vi "Decimate mixed channels data (Theo).vi"(9 "Selected Waveform":enum16{"Left graph", "Right graph"}(ring)=enum."Right graph", 10 "waveform":waveform(dbl)={"t0"=timestamp(0 s since 1904-01-01), "dt"=1e-06, "Y"=[]}) -> (0 "multiple tone information":T1(array[cluster])=[{"detected frequency"=59.40457132494078, "detected amplitude"=677.5224683183739, "detected phase (deg)"=-6.85916777032908}, {"detected frequency"=10023.302847711435, "detected amplitude"=302.0949374874943, "detected phase (deg)"=265.4481634375171}, {"detected frequency"=20019.602268100927, "detected amplitude"=136.99007273675608, "detected phase (deg)"=123.98051462950585}, {"detected frequency"=30006.01918128676, "detected amplitude"=20.477000538882503, "detected phase (deg)"=-16.173557072223005}] {"detected phase (deg)" format="%_6g"; "detected amplitude" format="%_6p"; "detected frequency" format="%_6p"}, 2 "output waveform":waveform(dbl))   [LabVIEW 2017]
uses:
  <vilib>/measure/NI_MAPro.lvlib
  <vilib>/express/express analysis/Spectral/XNode/ExpressSpectralMeasurementsBlockNode.xnode
  <vilib>/express/express analysis/Spectral/Block/exnSpectralBlock spectral measurements RMS poly.vi
  <vilib>/express/express analysis/Spectral/Block/exnSpectralBlock spectral measurements RMS WFM.vi
  <vilib>/measure/matone.llb/Extract Multiple Tone Information 1 Chan.vi
panel:
  out "Phase":cluster{"f0":dbl, "df":dbl, "phase":dbl[]}
  out "Measurement Output":cluster{"f0":dbl, "df":dbl, "magnitude":dbl[]}
  in  "Paste copied Excel data column in this box":string="442\n58\n454\n60\n425\n59\n424\n63\n423\n64\n371\n59\n492\n63\n416\n60\n390\n63\n393\n64\n472\n60\n457\n59\n461\n61\n383\n62\n415\n61\n416\n59\n421\n61\n430\n60\n440\n63\n429\n55\n407\n60\n479\n63\n463\n64\n389\n54\n449\n65\n443\n61\n415\n61\n419\n62\n396\n61\n379\n56\n386\n60\n404\n69\n349\n62\n466\n58\n450\n62\n414\n57\n433\n61\n477\n63\n397\n60\n402\n58\n457\n59\n466\n61\n445\n60\n416\n62\n459\n65\n464\n65\n441\n62\n408\n63\n437\n57\n388\n60\n429\n65\n445\n55\n460\n66\n419\n60\n431\n59\n450\n64\n451\n60\n435\n63\n431\n61\n450\n62\n423\n60\n423\n61\n434\n62\n454\n65\n417\n65\n403\n58\n462\n57\n430\n56\n451\n56\n431\n59\n384\n56\n462\n66\n476\n59\n436\n62\n460\n64\n467\n60\n430\n55\n411\n56\n498\n61\n426\n68\n469\n66\n445\n56\n428\n55\n455\n62\n447\n59\n407\n6..."
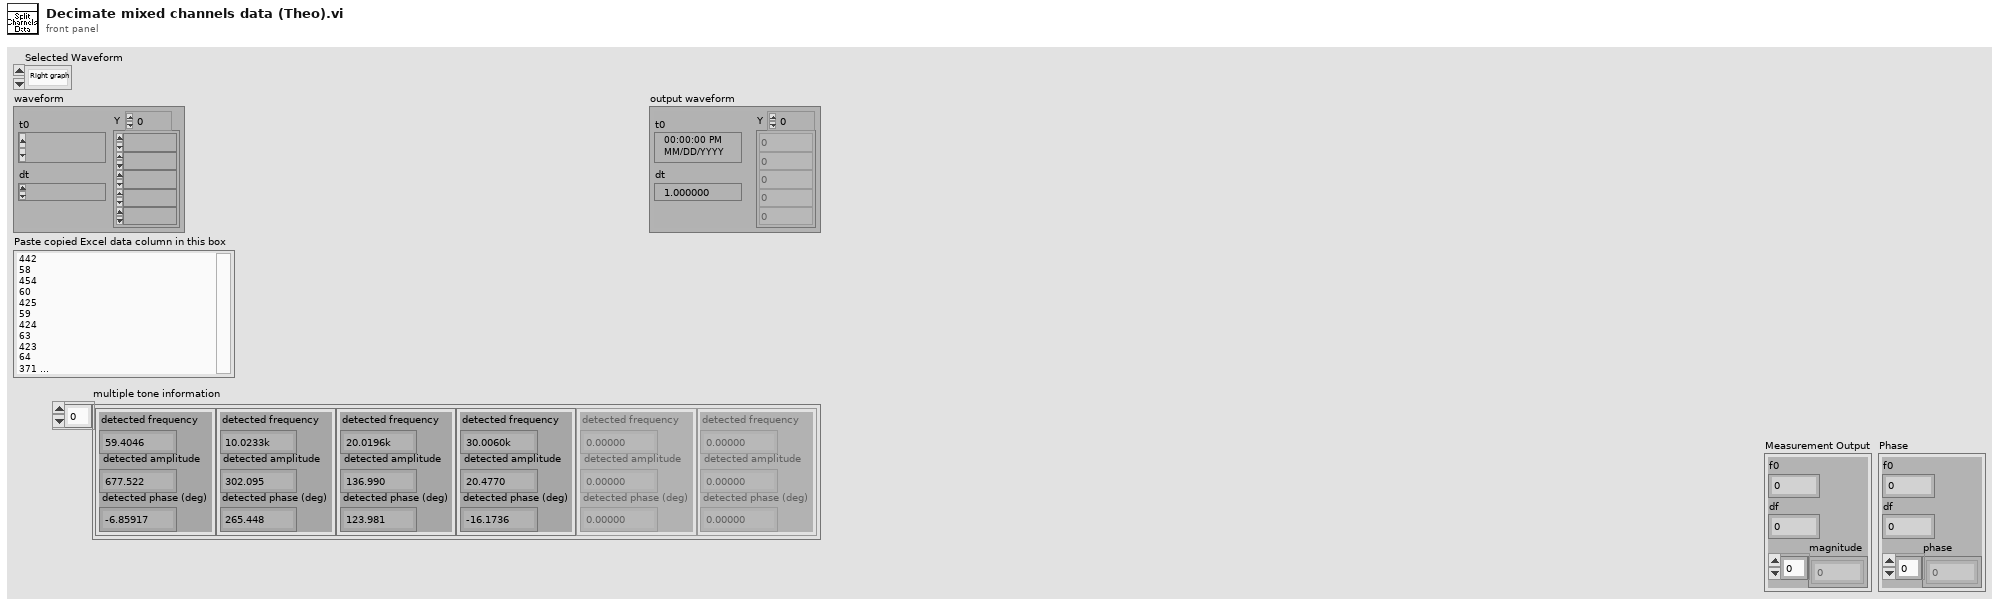
[diagram p1: front panel]
types:
  T1 = cluster{"detected frequency":dbl, "detected amplitude":dbl, "detected phase (deg)":dbl}[]
  T2 = enum32{"none", "input signal", "detected signal", "residual signal"}
  T3 = cluster{"averaging mode":u16, "weighting mode":u16, "number of averages":u32}
  T4 = cluster{"dB On (F)":bool, "unwrap phase (F)":bool, "convert to degree (F)":bool}
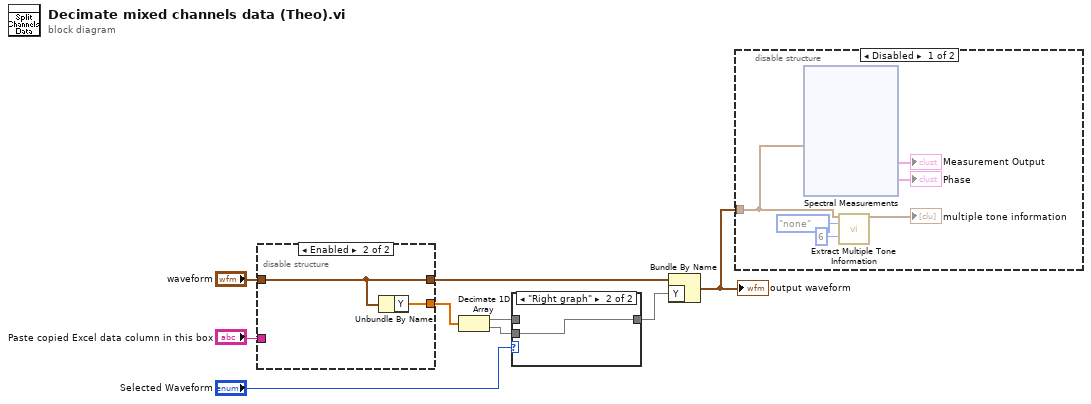
[diagram p0: block diagram]
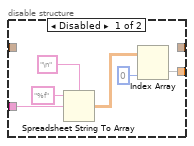
[diagram p4: hidden frame]
diagram:
  n1 = disable-structure shown="Enabled" {
    disable-tunnel: "Paste copied Excel data column in this box" -> [w15 _]
    disable-tunnel: [w10 w17] -> w8
    disable-tunnel: "waveform" -> [_ w16]
    disable-tunnel: [_ w16] -> w5
    frame Disabled {
      n2 = Spreadsheet String To Array(delimiter (Tab)="\n", format string="%f", spreadsheet string=w15) -> (array=w12:dbl[][])  [unwired: 1 in]
      n3 = Index Array(array=w12, index (col)=0 ("disabled index (col)")) -> (element=w10:dbl[])  [unwired: 1 in]
    }
    frame Enabled {
      n4 = Unbundle By Name(w16) -> ("Y"=w17:dbl[])
    }
  }
  n5 = Decimate 1D Array(w8) -> (w4:dbl[], w2:dbl[])
  n6 = case shown="\"Right graph\"" "Selected Waveform" {
    tunnel: w4 -> [w18 _]
    tunnel: [w18 w19] -> w3
    tunnel: w2 -> [_ w19]
    frame "Left graph", Default {
    }
    frame "Right graph" {
    }
  }
  n7 = Bundle By Name ("Build Waveform")(cluster=w5, "Y"=w3) -> (w7:waveform(dbl))
  "output waveform" <- w7
  n8 = disable-structure shown="Disabled" {
    disable-tunnel: w7 -> [w22 _]
    frame Disabled {
      n9 = xnode "Spectral Measurements"("Signals"=w22) -> ("Measurement Output"=→"Measurement Output":cluster{"f0":dbl, "df":dbl, "magnitude":dbl[]}, "Phase"=→"Phase":cluster{"f0":dbl, "df":dbl, "phase":dbl[]})  [unwired: 1 in, 1 out]
      n10 = call-poly <vilib>:"Extract Multiple Tone Information.vi"("time signal in"=w22, "export mode"=T2."none", "max num tones"=6) -> ("multiple tone information"=→"multiple tone information":T1)  [unwired: 10 in, 2 out]
    }
    frame Enabled {
    }
  }
